vi "手动打印界面.vi"() -> ()   [LabVIEW 2018]
uses:
  <vilib>/Utility/miscctls.llb/LVDateTimeRec.ctl
  <vilib>/ProgressBar/Progress Bar Dialog.lvclass
panel:
  in  "日":i32=1 min=1 max=31
  in  "月":i32=1 min=1 max=12
  in  "年":i32=1900 min=1900 max=3000
  in  "退出":bool
  in  "打印":bool
  in  "选择班次":string(combo)
  in  "型号选择":string(combo)
  in  "起始流水号":i32
  in  "打印个数":i32
  in  "选择灯件左/右":enum32{"单选选项1", "单选选项2"}(radio)
  # "时间"
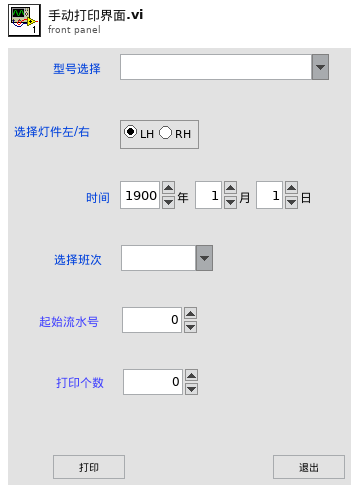
[diagram p1: front panel]
types:
  T1 = typedef "LVDateTimeRec.ctl" = cluster{"秒数的小数部分":dbl, "秒":i32, "分":i32, "时":i32, "日":i32, "月":i32, "年":i32, "天数（周）":i32, "天数（年）":i32, "DST":i32}
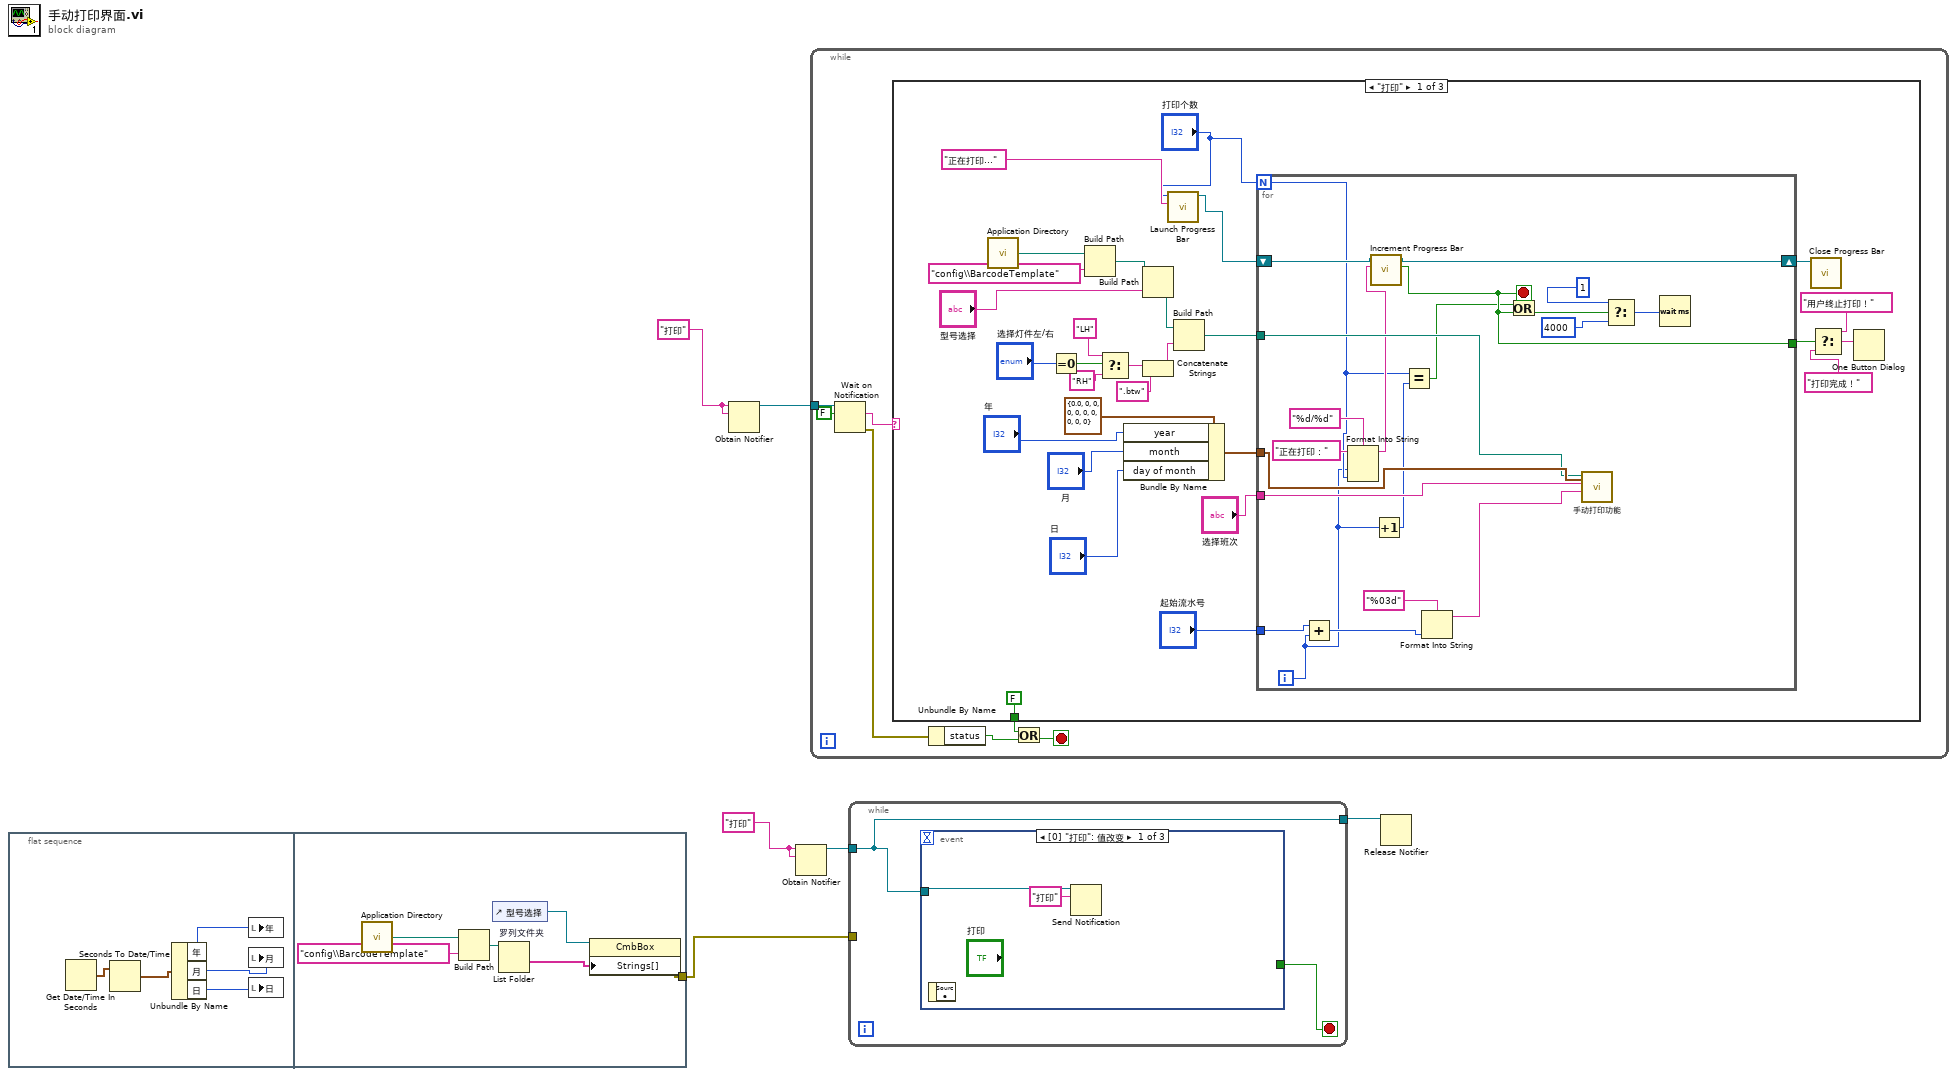
[diagram p0: block diagram]
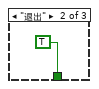
[diagram p2: hidden frame]
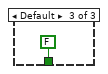
[diagram p3: hidden frame]
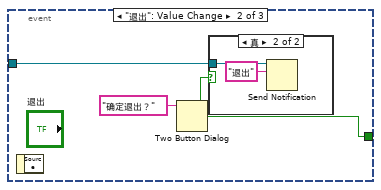
[diagram p4: hidden frame]
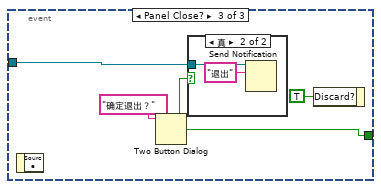
[diagram p6: hidden frame]
diagram:
  w4 = "打印" ("名称（未命名）")
  w6 = "打印" ("名称（未命名）")
  n1 = flat-sequence {
    tunnel: [w12] -> w1
    frame #0 {
      n2 = Get Date/Time In Seconds() -> (seconds since 1Jan1904=w11:timestamp)
      n3 = Seconds To Date/Time(time stamp (now)=w11) -> (date time rec=w10:T1)  [unwired: 1 in]
      n4 = Unbundle By Name(w10) -> ("年"=w9:i32, "月"=w8:i32, "日"=w7:i32)
      n5 = local write "年"(w9) -> ()
      n6 = local write "月"(w8) -> ()
      n7 = local write "日"(w7) -> ()
    }
    frame #1 {
      n8 = call <vilib>:"Application Directory.vi"() -> ("Application Directory"=w14:path)
      n9 = Build Path(base path=w14, name or relative path="config\\BarcodeTemplate" ("名称或相对路径")) -> (appended path=w15:path)
      n10 = control-ref of="型号选择"() -> (w17:refnum<vi>)
      n11 = List Folder "罗列文件夹"(path=w15) -> (folder names=w16:string[])  [unwired: 3 in, 3 out]
      n12 = property class="CmbBox"(reference=w17, "Strings[]"=w16) -> (error out=w12:errorcluster)  [unwired: 1 in, 1 out]
    }
  }
  n13 = Obtain Notifier(name (unnamed)=w4, notification data type=w4) -> (notifier out=w3:refnum<notifier>)  [unwired: 2 in, 2 out]
  n14 = Obtain Notifier(name (unnamed)=w6, notification data type=w6) -> (notifier out=w5:refnum<notifier>)  [unwired: 2 in, 2 out]
  n15 = while {
    tunnel: w3 -> [w24]
    stop <- w21 stop-if-true
    n16 = Wait on Notification(notifier=w24, ignore previous (F)=FALSE ("忽略上一个(F)")) -> (notification=w23:string, error out=w20:errorcluster)  [unwired: 2 in, 2 out]
    n17 = case shown="\"打印\"" w23 {
      tunnel: [FALSE ("x") TRUE ("x") FALSE ("x")] -> w19
      frame "打印" {
        n18 = call <vilib>:"Application Directory.vi"() -> ("Application Directory"=w45:path)
        n19 = Equal To 0?(x="选择灯件左/右") -> (x = 0?=w39:bool)
        n20 = Build Path(base path=w45, name or relative path="config\\BarcodeTemplate" ("名称或相对路径")) -> (appended path=w43:path)
        n21 = Select(t="LH" ("名称（未命名）"), s=w39, f="RH" ("名称（未命名）")) -> (s? t:f=w36:string)
        n22 = Bundle By Name(cluster=T1 {"fractional second"=0.0, "second"=0, "minute"=0, "hour"=0, "day of month"=0, "month"=0, "year"=0, "day of week"=0, "day of year"=0, "DST"=0} ("日期时间记录"), "year"="年", "month"="月", "day of month"="日") -> (w49:T1)
        n23 = Build Path(base path=w43, name or relative path="型号选择") -> (appended path=w41:path)
        n24 = Concatenate Strings(w36, ".btw" ("字符串")) -> (w26:string)
        n25 = call <vilib>:"Launch Progress Bar.vi"("Main Title (\"Working...\")"="正在打印..." ("Window Title (Progress)"), "Total Count"="打印个数") -> ("Progress Bar Dialog"=w32:refnum<class "Progress Bar Dialog.lvclass">)  [unwired: 8 in, 1 out]
        n26 = Build Path(base path=w41, name or relative path=w26) -> (appended path=w35:path)
        n27 = for {
          N: "打印个数" -> [w57]
          shift-right: [w64] -> w31
          shift-left: w32 -> [w65]
          tunnel: "起始流水号" -> [w72]
          tunnel: "选择班次" -> [w71]
          tunnel: w49 -> [w68]
          tunnel: w35 -> [w67]
          tunnel: [w63] -> w29
          i -> [w56]
          stop <- w63 stop-if-true
          n28 = Add(x=w72, y=w56) -> (x+y=w66:i32)
          n29 = Format Into String(format string="%d/%d" ("格式字符串"), initial string="正在打印：" ("初始字符串"), w56, w57) -> (resulting string=w59:string)  [unwired: 1 in, 1 out]
          n30 = call <vilib>:"Increment Progress Bar.vi"("Step Name (\"\")"=w59, "Progress Bar Dialog in"=w65) -> ("Cancelled?"=w63:bool, "Progress Bar Dialog out"=w64:refnum<class "Progress Bar Dialog.lvclass">)  [unwired: 7 in, 1 out]
          n31 = Increment(x=w56) -> (x+1=w54:i32)
          n32 = Equal?(x=w57, y=w54) -> (x = y?=w55:bool)
          n33 = Format Into String(format string="%03d" ("格式字符串"), w66) -> (resulting string=w69:string)  [unwired: 2 in, 1 out]
          n34 = Or(x=w55, y=w63) -> (x .or. y?=w58:bool)
          n35 = call "手动打印功能.vi"("日期时间记录"=w68, "流水号（3位）"=w69, "班次"=w71, "路径"=w67) -> ()  [unwired: 6 in, 2 out]
          n36 = Select(t=u32 1 ("等待时间（毫秒）"), s=w58, f=u32 4000 ("等待时间（毫秒）")) -> (s? t:f=w62:u32)
          n37 = Wait (ms)(milliseconds to wait=w62) -> ()  [unwired: 1 out]
        }
        n38 = call <vilib>:"Close Progress Bar.vi"("Progress Bar Dialog"=w31) -> ()  [unwired: 10 in, 1 out]
        n39 = Select(t="用户终止打印！" ("名称（未命名）"), s=w29, f="打印完成！" ("名称（未命名）")) -> (s? t:f=w30:string)
        n40 = One Button Dialog(message=w30) -> ()  [unwired: 1 in, 1 out]
      }
      frame "退出" {
      }
      frame Default {
      }
    }
    n41 = Unbundle By Name(w20) -> ("status"=w22:bool)
    n42 = Or(x=w19, y=w22) -> (x .or. y?=w21:bool)
  }
  n43 = while {
    tunnel: w5 -> [w77]
    tunnel: [w77] -> w2
    tunnel: w1 -> [_]
    stop <- w78 stop-if-true
    n44 = event shown="[0] \"打印\": 值改变" {
      selector: _ -> [_ _ _]
      dyn-events: _ -> [_ _ _]
      timeout: _ -> [_ _ _]
      tunnel: [_ w82 w88] -> w78
      tunnel: w77 -> [w80 w81 w87]
      event "打印": Value Change {
        n45 = event-data() -> ()  [unwired: 1 in, 1 out]
        n46 = Send Notification(notification="打印" ("通知"), notifier=w80) -> ()  [unwired: 1 in, 2 out]
      }
      event "退出": Value Change {
        n47 = event-data() -> ()  [unwired: 1 in, 1 out]
        n48 = Two Button Dialog(message="确定退出？" ("消息")) -> (T button?=w82:bool)  [unwired: 2 in]
        n49 = case shown="真" w82 {
          tunnel: w81 -> [_ w85]
          frame False {
          }
          frame True {
            n50 = Send Notification(notification="退出" ("通知"), notifier=w85) -> ()  [unwired: 1 in, 2 out]
          }
        }
      }
      event Panel Close? {
        n51 = event-data() -> ()  [unwired: 1 in, 1 out]
        n52 = Two Button Dialog(message="确定退出？" ("消息")) -> (T button?=w88:bool)  [unwired: 2 in]
        n53 = case shown="真" w88 {
          tunnel: w87 -> [_ w91]
          frame False {
          }
          frame True {
            n54 = Send Notification(notification="退出" ("通知"), notifier=w91) -> ()  [unwired: 1 in, 2 out]
          }
        }
        n55 = event-data("Discard?"=TRUE ("放弃？")) -> ()  [unwired: 1 in, 1 out]
      }
    }
  }
  n56 = Release Notifier(notifier=w2) -> ()  [unwired: 2 in, 3 out]
